vi "Active Read.vi"(4 "error in (no error)":errorcluster, 6 "Container State":T2, 7 "Display State In":T1) -> (0 "error out":errorcluster, 2 "Value":bool[](array[boolean]), 3 "Display State Out":T1)   [LabVIEW 2015, in "1D Buffer.xctl"]
uses:
  1D Buffer.xctl
  <vilib>/_xctls/Container State.ctl
  State.ctl
  <vilib>/_xctls/XControlSupport.lvlib
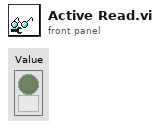
[diagram p1: front panel]
types:
  T1 = typedef "1D Buffer.xctl/State.ctl" = cluster{"Data Array":sgl[][], "Time Array":timestamp[], "History":u16, "Variable":bool[], "Plot Details":cluster{"Name":string, "Line Width":u8, "Line Style":u8, "Color":u32}[], "Y-Axis Labels":string[], "legend visible":bool}
  T2 = typedef "XControlSupport.lvlib/Container State.ctl" = cluster{"Indicator?":bool, "Run Mode?":bool, " Refnum":refnum<vi>}
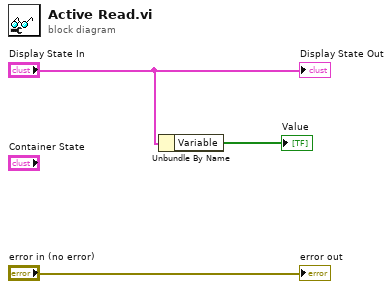
[diagram p0: block diagram]
diagram:
  n1 = Unbundle By Name("Display State In") -> ("Variable"=→"Value":bool[])
  "error out" <- "error in (no error)"
  "Display State Out" <- "Display State In"
